vi "Configure Trigger Source [TRG].vi"(8 "error in (no error)":errorcluster, 9 "trigger source (External)":i32(ring)=1 items=["Internal"=3, "External"=1, "Software Trigger Function"=2, "PXI TRIG0 or VXI TTL0"=111, "PXI TRIG1 or VXI TTL1"=112, "PXI TRIG2 or VXI TTL2"=113, "PXI TRIG3 or VXI TTL3"=114, "PXI TRIG4 or VXI TTL4"=115, "PXI TRIG5 or VXI TTL5"=116, "PXI TRIG6 or VXI TTL6"=117, "PXI TRIG7 or VXI TTL7"=118, "ECL0"=119, "ECL1"=120, "PXI Star"=131, "RTSI 0"=141, "RTSI 1"=142, "RTSI 2"=143, "RTSI 3"=144, "RTSI 4"=145, "RTSI 5"=146, "RTSI 6"=147], 10 "channel name (\"CHANNEL1\")":string="CHANNEL1", 11 "CS++Fgen in":refnum<class "CS++Fgen.lvclass">) -> (0 "error out":errorcluster, 3 "CS++Fgen out":refnum<class "CS++Fgen.lvclass">)   [LabVIEW 2013, in "CS++Fgen.lvlib" / "CS++Fgen.lvclass"]
doc: "This VI configures the trigger source for a channel.\n\nNotes:\n\n(1) This VI is part of the IviFgenTrigger [TRG] extension group."
uses:
  CS++Fgen.lvclass
  CSPP_Core/Classes/CS++ProcessVariables/ProcessVariable/PV.lvclass
  PV-Enum-n.ctl
  CSPP_Core/Classes/CS++ProcessVariables/ProcessVariable/PV.lvclass/PV.ctl
  CS++Fgen.lvclass/CS++Fgen.ctl
  CSPP_Core/Classes/CS++ProcessVariables/PVConnection/PVConnection.lvclass
  CSPP_Core/Classes/CS++ProcessVariables/ProcessVariable/Write Data.vi
  CSPP_Core/Classes/CS++ProcessVariables/ProcessVariable/Write Timestamp.vi
  CSPP_Core/Classes/CS++ProcessVariables/ProcessVariable/Write Quality.vi
  CSPP_Core/Classes/CS++ProcessVariables/ProcessVariable/Write status.vi
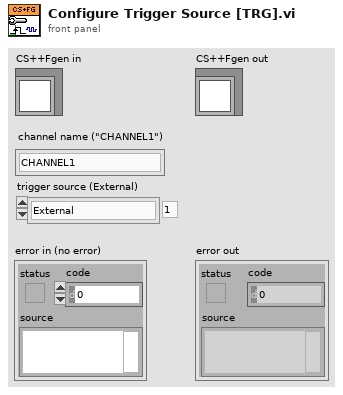
[diagram p1: front panel]
types:
  T1 = typedef "CS++Fgen.lvlib/CS++Fgen.lvclass/PV-Enum-n.ctl" = enum16{"Amplitude", "Arb-Frequency", "DCOffset", "Frequency", "OutputImpedance", "StartPhase", "AdvancedTriggerSlope", "AM-Source", "BurstCount", "FM-Source", "OperationMode", "ResumeTriggerSlope", "StartTriggerSlope", "StopTriggerSlope", "Waveform", "AM-Enabled", "ChannelEnabled", "FM-Enabled", "AdvancedTriggerSource", "ResumeTriggerSource", "StartTriggerSource", "StopTriggerSource", "TriggerSource"}
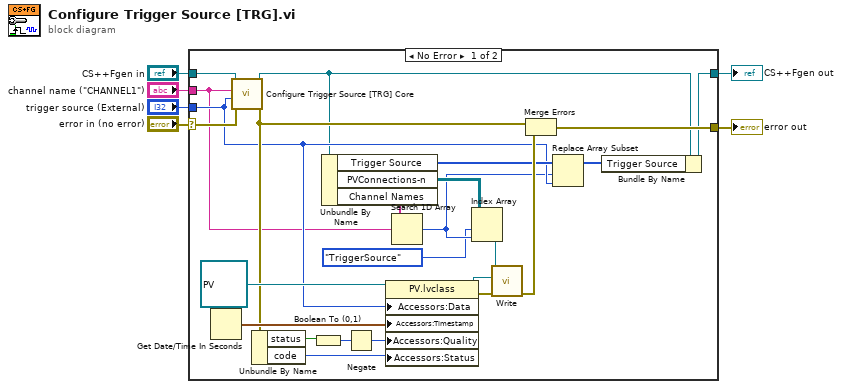
[diagram p0: block diagram]
diagram:
  n1 = case shown="No Error" "error in (no error)" {
    selector: "error in (no error)" -> [w29 w32]
    tunnel: [w14 w32] -> w5
    tunnel: [w9 w31] -> w3
    tunnel: "CS++Fgen in" -> [w30 w31]
    tunnel: "channel name (\"CHANNEL1\")" -> [w11 _]
    tunnel: "trigger source (External)" -> [w12 _]
    frame No Error {
      n2 = Get Date/Time In Seconds() -> (seconds since 1Jan1904=w28:timestamp)
      n3 = call-dynamic "Configure Trigger Source [TRG] Core.vi"("error in (no error)"=w29, "trigger source (External)"=w12, "channel name (\"CHANNEL1\")"=w11, "CS++Fgen in"=w30) -> ("error out"=w13:errorcluster, "CS++Fgen out"=w10:refnum<class "CS++Fgen.lvclass">)  [unwired: 6 in]
      n4 = Unbundle By Name(w13) -> ("status"=w20:bool, "code"=w18:i32)
      n5 = Boolean To (0,1)(Boolean=w20) -> (0, 1=w19:i16)
      n6 = Unbundle By Name(w10) -> ("Trigger Source"=w16:i32[], "PVConnections-n"=w23:refnum<class "PVConnection.lvclass">[][], "Channel Names"=w24:string[])
      n7 = Negate(x=w19) -> (-x=w17:i16)
      n8 = property class="PV.lvclass"(reference=refnum<class "PV.lvclass"> refnum ("PV"), "Accessors:Data"=w12, "Accessors:Timestamp"=w28, "Accessors:Quality"=w17, "Accessors:Status"=w18) -> (reference out=w25:refnum<class "PV.lvclass">, error out=w26:errorcluster)  [unwired: 1 in]
      n9 = Search 1D Array(1D array=w24, element=w11) -> (index of element=w8:i32)  [unwired: 1 in]
      n10 = Index Array(array=w23, index (row)=PV-Enum-n."TriggerSource" ("PV-Enum-n"), index (col)=w8) -> (element=w22:refnum<class "PVConnection.lvclass">)
      n11 = call-dynamic "Write.vi"("error in (no error)"=w26, "PV"=w25, "PVConnection in"=w22) -> ("error out"=w21:errorcluster)  [unwired: 7 in, 1 out]
      n12 = Merge Errors(w13, w21) -> (w14:errorcluster)
      n13 = Replace Array Subset(array=w16, new element=w12, index=w8) -> (w15:i32[])
      n14 = Bundle By Name(cluster=w10, "Trigger Source"=w15) -> (w9:refnum<class "CS++Fgen.lvclass">)
    }
    frame Error {
    }
  }
  "error out" <- w5
  "CS++Fgen out" <- w3
